vi "Format Tree.vi"(8 "error in (no error)":errorcluster, 10 "Tag":string, 11 "Test Executive Builder View in":refnum<class "Test Executive Builder View.lvclass">) -> (0 "error out":errorcluster, 3 "Test Executive Builder View out":refnum<class "Test Executive Builder View.lvclass">)   [LabVIEW 2017, in "Test Executive Builder View.lvclass"]
uses:
  <vilib>/gpm_packages/@cs/Test-executive-builder/Source/Test Executive Builder View/Test Executive Builder View/Test Executive Builder View.lvclass
  <vilib>/gpm_packages/@cs/Test-executive-builder/Source/Test Executive Builder View/Test Executive Builder View/Test Executive Builder View.lvclass/Test Executive Builder View.ctl
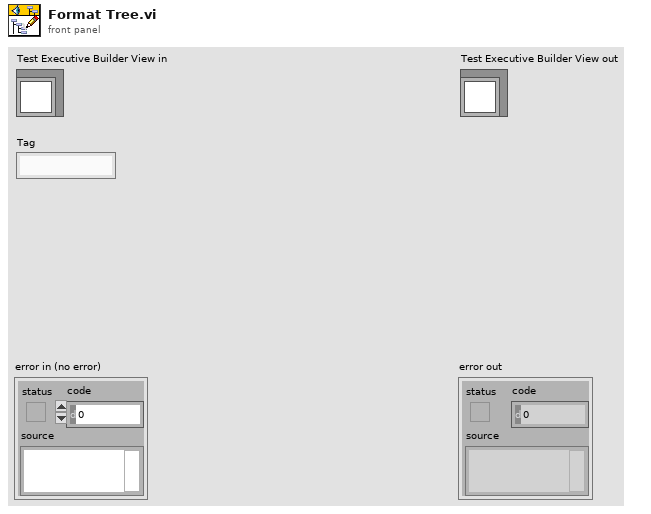
[diagram p1: front panel]
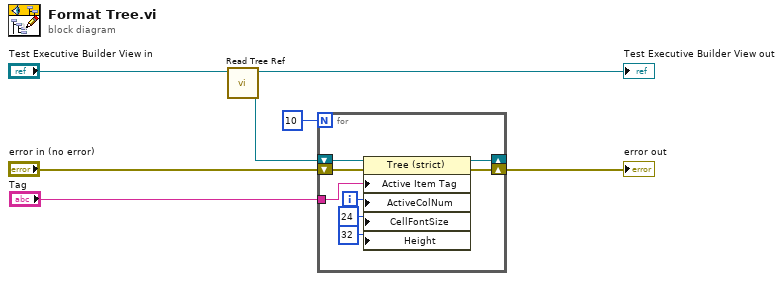
[diagram p0: block diagram]
diagram:
  n1 = call <vilib>:"Read Tree Ref.vi"("Test Executive Builder View in"="Test Executive Builder View in") -> ("Tree Ref"=w2:refnum<vi>, "Test Executive Builder View out"=→"Test Executive Builder View out":refnum<class "Test Executive Builder View.lvclass">)  [unwired: 9 in]
  n2 = for {
    N: 10 -> [_]
    shift-right: [w14] -> _
    shift-left: w2 -> [w15]
    shift-right: [w12] -> w5
    shift-left: "error in (no error)" -> [w13]
    tunnel: "Tag" -> [w10]
    i -> [w11]
    n3 = property class="Tree (strict)"(reference=w15, error in=w13, "Active Item Tag"=w10, "ActiveColNum"=w11, "CellFontSize"=u32 24 ("Active Cell:Cell Font:Size"), "Height"=32 ("Active Cell:Cell Size:Height")) -> (reference out=w14:refnum<vi>, error out=w12:errorcluster)
  }
  "error out" <- w5
